vi "Send funct data re-process event.vi"(8 "error in (no error)":errorcluster, 11 "Waveform Graph in":T1) -> (0 "error out":errorcluster)   [LabVIEW 2020]
uses:
  xcontrol/Typedefs/Xctrl-Waveform graph ref.ctl
  Typedefs/Registered event names enum.ctl
  xcontrol/XGrapher.xctl
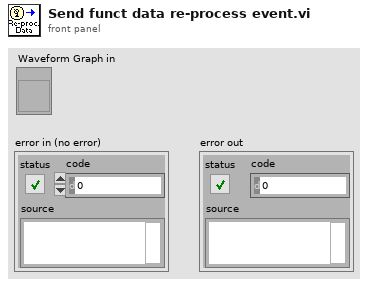
[diagram p1: front panel]
types:
  T1 = typedef "XGrapher.xctl/Xctrl-Waveform graph ref.ctl" = refnum<vi>
  T2 = typedef "Registered event names enum.ctl" = enum16{"Register", "Load dataset in funct viewer", "Re-process data", "Export selected ROI data-full"}
  T3 = typedef "LVRangeTypeDef.ctl" = cluster{"Minimum":dbl, "Maximum":dbl, "Increment":dbl, "Minor Increment":dbl, "Start":dbl}
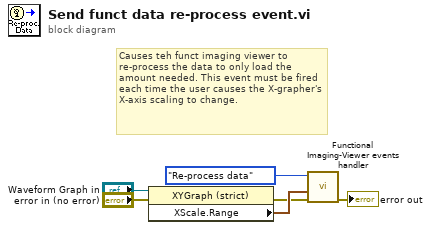
[diagram p0: block diagram]
diagram:
  # "Causes teh funct imaging viewer to re-process the data to only load the amount needed. This event must be fired each time the user causes the X-grapher's X-axis scaling to change."
  n1 = property class="XYGraph (strict)"(reference="Waveform Graph in", error in="error in (no error)") -> (error out=w3:errorcluster, "XScale.Range"=w4:T3)  [unwired: 1 out]
  n2 = call "Functional Imaging-Viewer events handler.vi"("error in (no error)"=w3, "NewRange"=w4, "Event Function"=Registered_event_names_enum."Re-process data") -> ("error out"=→"error out":errorcluster)  [unwired: 7 in, 1 out]
